vi "Return data.vi"(9 "Array Return":dbl[][](array[numeric]), 10 "Array Input":dbl[][](array[numeric]), 11 "Return":bool caption="Scan") -> (2 "Array out":dbl[][](array[numeric]))   [LabVIEW 2018]
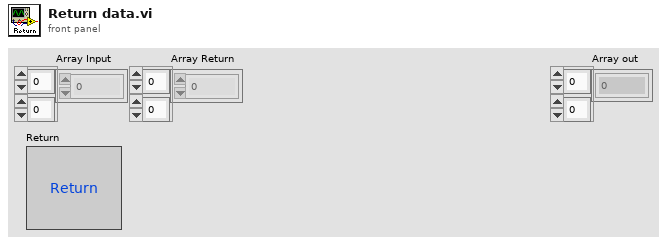
[diagram p1: front panel]
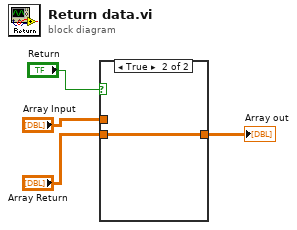
[diagram p0: block diagram]
diagram:
  n1 = case shown="True" "Return" {
    tunnel: "Array Input" -> [w5 _]
    tunnel: [w5 w6] -> w2
    tunnel: "Array Return" -> [_ w6]
    frame False {
    }
    frame True {
    }
  }
  "Array out" <- w2
